vi "Read blockDiagramRef.vi"(8 "error in (no error)":errorcluster, 11 "BlockDiagram In":refnum<class "BlockDiagram.lvclass">) -> (0 "error out":errorcluster, 2 "blockDiagramRef":refnum<vi>, 3 "BlockDiagram Out":refnum<class "BlockDiagram.lvclass">)   [LabVIEW 2023, in "TLC_Scripto.lvlib" / "BlockDiagram.lvclass"]
uses:
  BlockDiagram.lvclass
  C:/projects/TLC_Scripto/Source/GObject/GObject.lvclass
  GObject/Read ref.vi
  BlockDiagram.lvclass/BlockDiagram.ctl
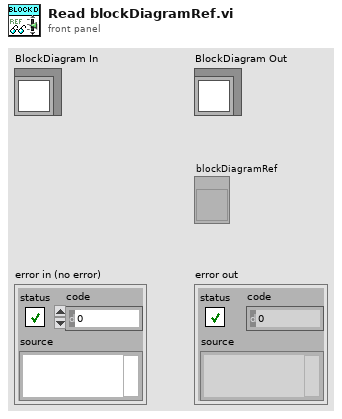
[diagram p1: front panel]
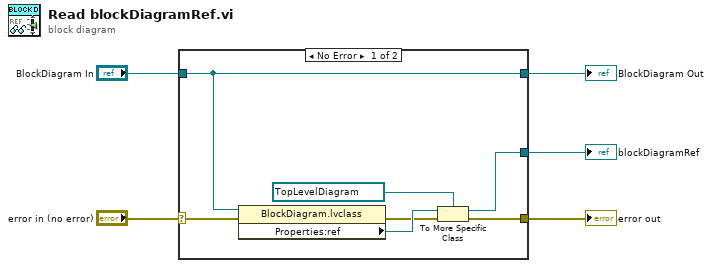
[diagram p0: block diagram]
diagram:
  n1 = case shown="No Error" "error in (no error)" {
    selector: "error in (no error)" -> [w8 w14]
    tunnel: [w10 w14] -> w4
    tunnel: [w12 w13] -> w2
    tunnel: "BlockDiagram In" -> [w12 w13]
    tunnel: [w9 _] -> w1
    frame No Error {
      n2 = property class="BlockDiagram.lvclass"(reference=w12, error in=w8) -> (error out=w7:errorcluster, "Properties:ref"=w11:refnum<vi>)  [unwired: 1 out]
      n3 = To More Specific Class(target class=refnum<vi> refnum ("Reference to Diagram"), reference=w11, error in=w7) -> (specific class reference=w9:refnum<vi>, error out=w10:errorcluster)
    }
    frame Error {
    }
  }
  "error out" <- w4
  "BlockDiagram Out" <- w2
  "blockDiagramRef" <- w1
